vi "Create NI 9422 - Digital Input.vi"(8 "error in":errorcluster, 11 "channel settings":T1[](array[typedef])) -> (0 "error out":errorcluster, 3 "NI 9422 out":refnum<class "NI 9422.lvclass">)   [LabVIEW 2020, in "Scan Engine Scripting.lvlib" / "NI 9422.lvclass"]
doc: "Creates and configures an instance of a NI-9422 digital input module that can be used to set a slot in a Scan Engine custom device chassis."
uses:
  NI 9422.lvclass
  Mode Classes/Controls/digital channel settings.ctl
  Mode Classes/Digital Input Mode/Digital Input Mode.lvclass
  C:/jenkins/workspace/ercat-custom-device_release_20.4/Custom Device Source/Scripting/Modules/Mode Classes/Mode/Mode.lvclass
  09133c77-b8c8-4b85-bcb4-a501a172f880.vi
  Scan Engine Scripting.lvlib
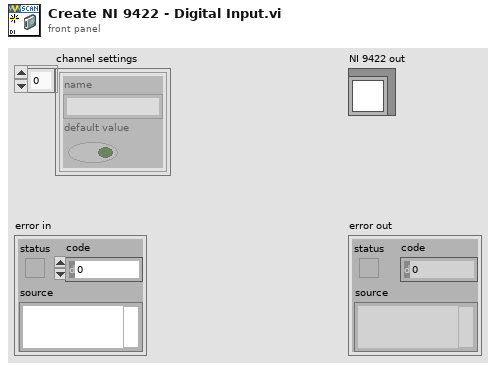
[diagram p1: front panel]
types:
  T1 = typedef "Scan Engine Scripting.lvlib/digital channel settings.ctl" = cluster{"name":string, "default value":bool}
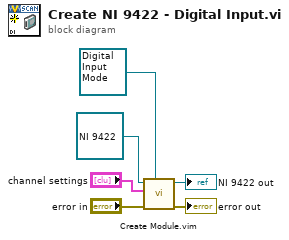
[diagram p0: block diagram]
diagram:
  n1 = call "Create Module.vim"("mode"=refnum<class "Digital Input Mode.lvclass"> refnum ("Scan Engine Scripting.lvlib:Digital Input Mode.lvclass"), "error in"="error in", "channel settings"="channel settings", "module in"=refnum<class "NI 9422.lvclass"> refnum ("NI 9422 in")) -> ("error out"=→"error out":errorcluster, "module out"=→"NI 9422 out":refnum<class "NI 9422.lvclass">)  [unwired: 6 in]
